vi "Parse Path String.vi"(0 "Path in":string, 2 "String Separator (:)":string=":") -> (4 "Folder Hierarchy":string[](array[string]), 5 "File/Folder":string)   [LabVIEW 2021, in "Strings.lvlib"]
doc: "Finds the last component of a path string."
uses:
  Strings.lvlib
  <userlib>/_OpenG.lib/string/string.llb/openg_string.lvlib
panel:
  # "see the AlliGator License on the block diagram (Ctrl+E or Window:Show Block Diagram)"
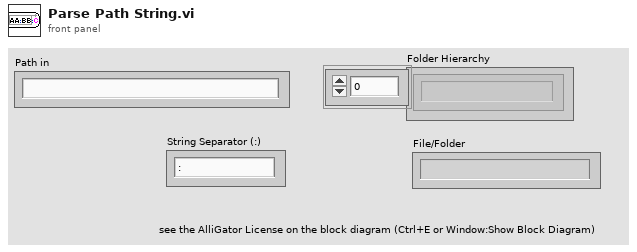
[diagram p1: front panel]
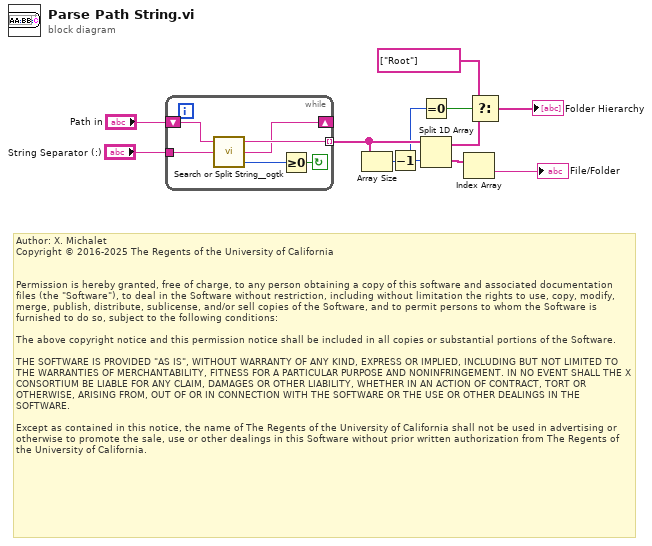
[diagram p0: block diagram]
diagram:
  # "Author: X. Michalet\nCopyright © 2016-2025 The Regents of the University of California\n \n\nPermission is hereby granted, free of charge, to any person obtaining a copy of this software and associated documentation files (the \"Software\"), to deal in the Software without restriction, including without limitation the rights to use, copy, modify, merge, publish, distribute, sublicense, and/or sell copies of the Software, and to permit persons to whom the Software is furnished to do so, subject to the following conditions:\n\nThe above copyright notice and this permission notice shall be included in all copies or substantial portions of the Software.\n\nTHE SOFTWARE IS PROVIDED \"AS IS\", WITHOUT WARRANTY OF ANY KIND, EXPRESS OR IMPLIED, INCLUDING BUT NOT LIMITED TO THE WARRANTIES OF MERCHANTABILITY, FITNESS FOR A PARTICULAR PURPOSE AND NONINFRINGEMENT. IN NO EVENT SHALL THE X CONSORTIUM BE LIABLE FOR ANY CLAIM, DAMAGES OR OTHER LIABILITY, WHETHER IN AN ACTION OF CONTRACT, TORT OR OTHERWISE, ARISING FROM, OUT OF OR IN CONNECTION WITH THE SOFTWARE OR THE USE OR OTHER DEALINGS IN THE SOFTWARE.\n\nExcept as contained in this notice, the name of The Regents of the University of California shall not be used in advertising or otherwise to promote the sale, use or other dealings in this Software without prior written authorization from The Regents of the University of California."
  n1 = while {
    tunnel: "String Separator (:)" -> [w16]
    shift-right: [w12] -> _
    shift-left: "Path in" -> [w17]
    tunnel: [w14] -> w8 mode=indexing
    stop <- w13 continue-if-true
    n2 = call <userlib>:"Search or Split String__ogtk.vi"("search string/char (-)"=w16, "string"=w17) -> ("offset after match"=w15:i32, "substring after match"=w12:string, "substring before match"=w14:string)  [unwired: 1 in]
    n3 = Greater Or Equal To 0?(x=w15) -> (x >= 0?=w13:bool)
  }
  n4 = Array Size(array=w8) -> (size(s)=w9:i32)
  n5 = Decrement(x=w9) -> (x-1=w5:i32)
  n6 = Equal To 0?(x=w5) -> (x = 0?=w4:bool)
  n7 = Split 1D Array(array=w8, index=w5) -> (first subarray=w3:string[], second subarray=w6:string[])
  n8 = Index Array(array=w6) -> (element=→"File/Folder":string)  [unwired: 1 in]
  n9 = Select(t=string[] ["Root"], s=w4, f=w3) -> (s? t:f=→"Folder Hierarchy":string[])
